vi "baogao5.vi"() -> ()   [LabVIEW 2017]
panel:
  out "Histogram":dynamicdata(graph)
  in  "N":dbl
  out "k":i32
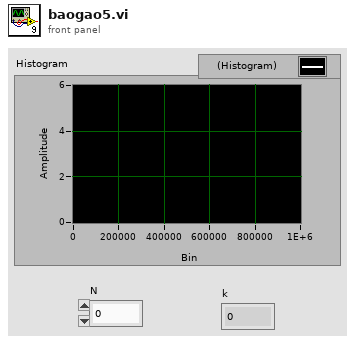
[diagram p1: front panel]
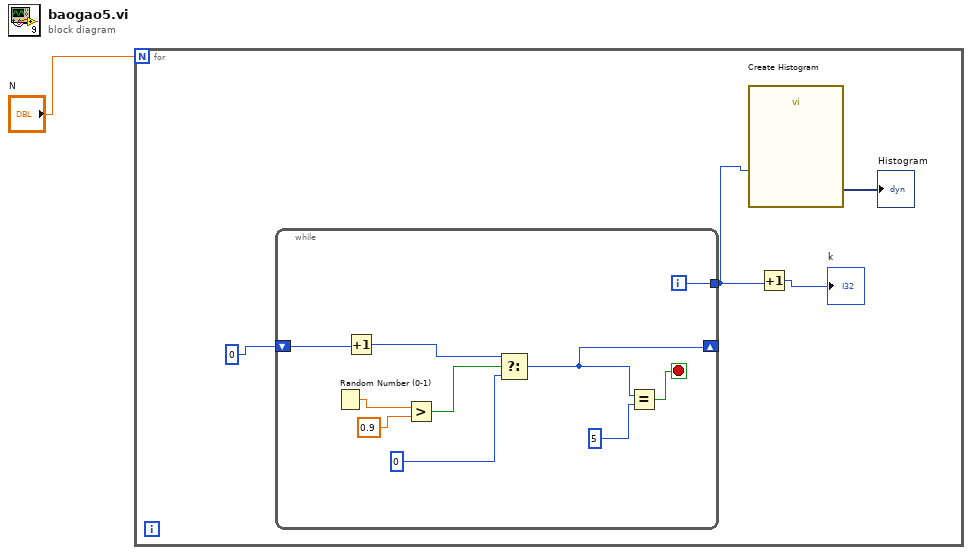
[diagram p0: block diagram]
diagram:
  n1 = for {
    N: "N" -> [_]
    n2 = while {
      tunnel: [w15] -> w3
      shift-right: [w6] -> _
      shift-left: 0 -> [w14]
      i -> [w15]
      stop <- w7 stop-if-true
      n3 = Random Number (0-1)() -> (number: 0 to 1=w12:dbl)
      n4 = Increment(x=w14) -> (x+1=w13:i32)
      n5 = Greater?(x=w12, y=0.9) -> (0:w10:bool)
      n6 = Select(t=w13, s=w10, f=0) -> (s? t:f=w6:i32)
      n7 = Equal?(x=w6, y=5) -> (x = y?=w7:bool)
    }
    n8 = call "Create Histogram"("Signal"=w3) -> ("Histogram"=→"Histogram":dynamicdata)  [unwired: 9 in, 1 out]
    n9 = Increment(x=w3) -> (x+1=→"k":i32)
  }
